vi "zc_jy.vi"(0 "action":string, 1 "LabVIEW Web Service Request":refnum<class "Web Request.lvclass"> caption="LabVIEW Web服务请求", 2 "jsren":string, 3 "sp_yijian":string, 5 "id":string, 7 "zc_luodi_num":string, 8 "sp_shuoming":string, 9 "zhriqi":string, 11 "didian":string, 12 "yongtu":string, 13 "shuoming":string, 14 "lc_num":string, 15 "key":string) -> (4 "error":errorcluster)   [LabVIEW 2017]
uses:
  <vilib>/wsapi/Web Request.lvclass
panel:
  in  "error 3":errorcluster={"status"=TRUE, "code"=255, "source"="当前资产不是“入库”状态！"} caption="error"
  out "postdata":string caption="post数据"
  out "error out":errorcluster caption="错误输出"
  # "Web服务请求输入接线端用于调用“Web服务”选板的VI。除非不需要访问该选板，否则不要在连线板上删除这个输入接线端。"
  # "添加至连线板的每一个其他输入控件，在URL中对应于一个输入。如需在接线端模式输出（默认设置）下包含显示控件，则该显示控件必须与连线板相连。"
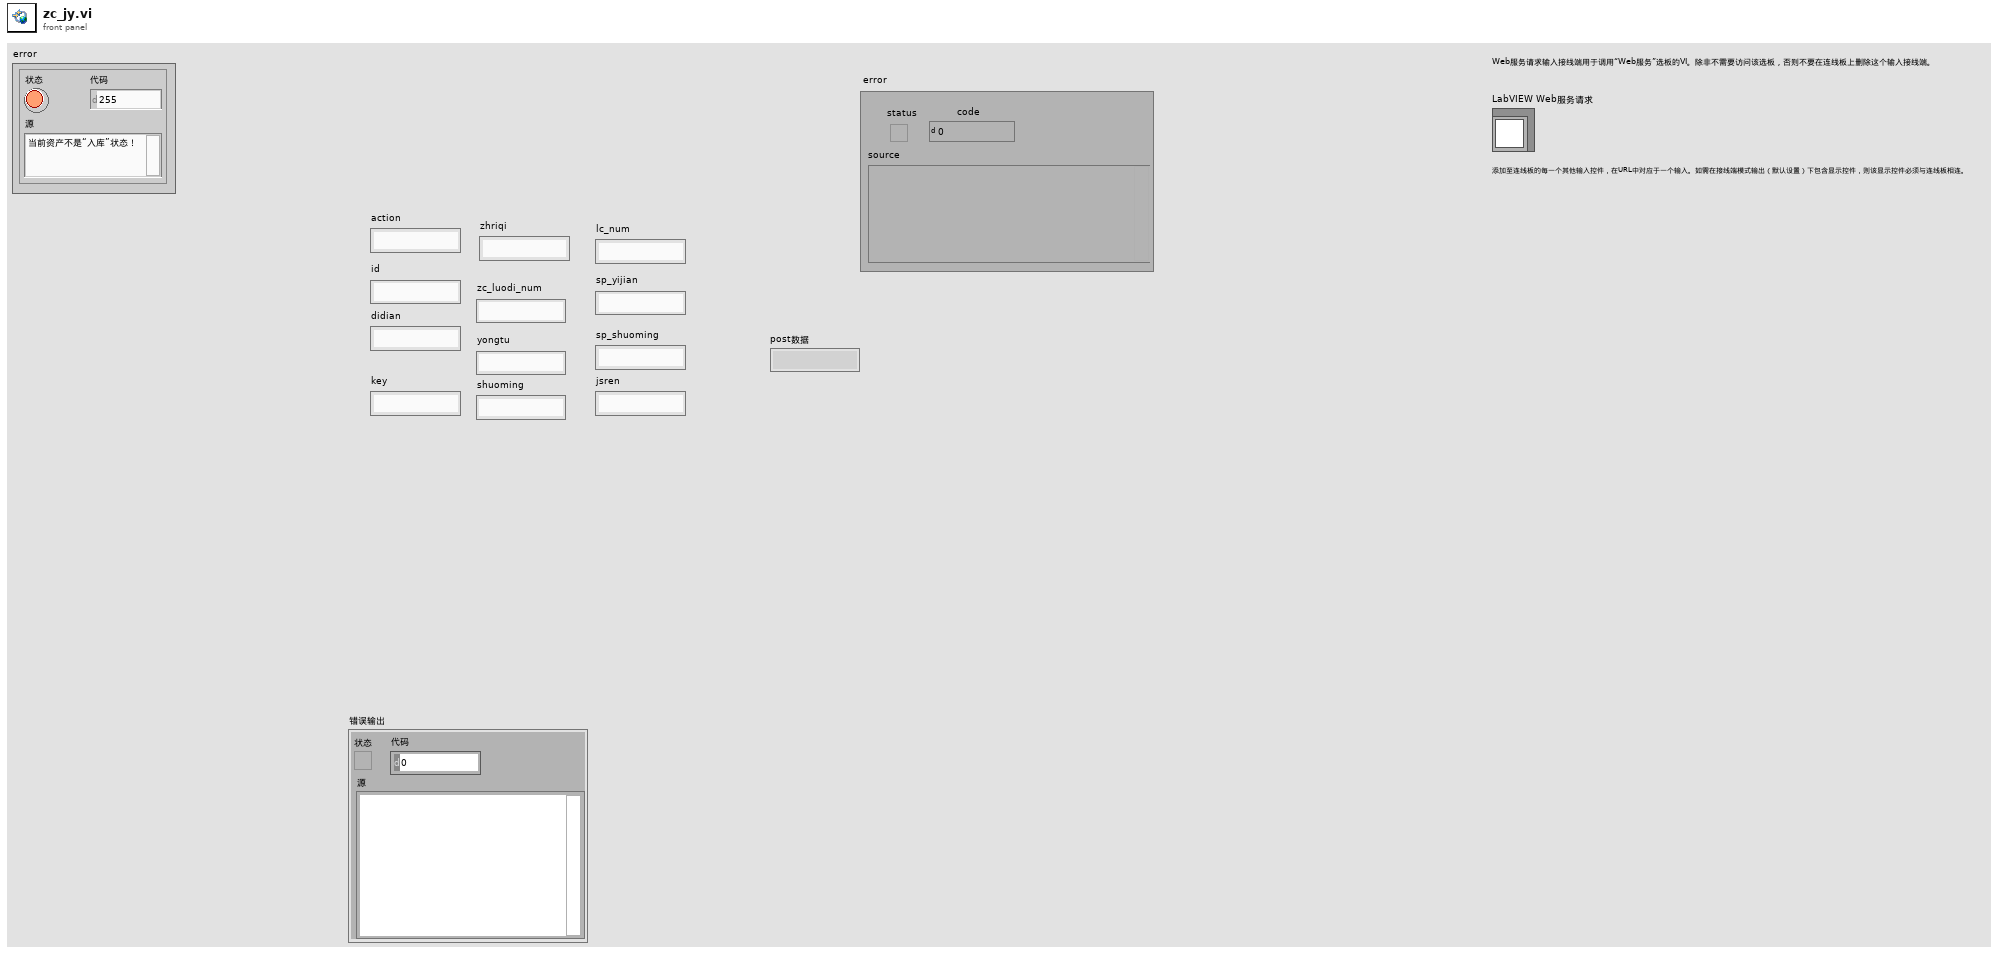
[diagram p1: front panel]
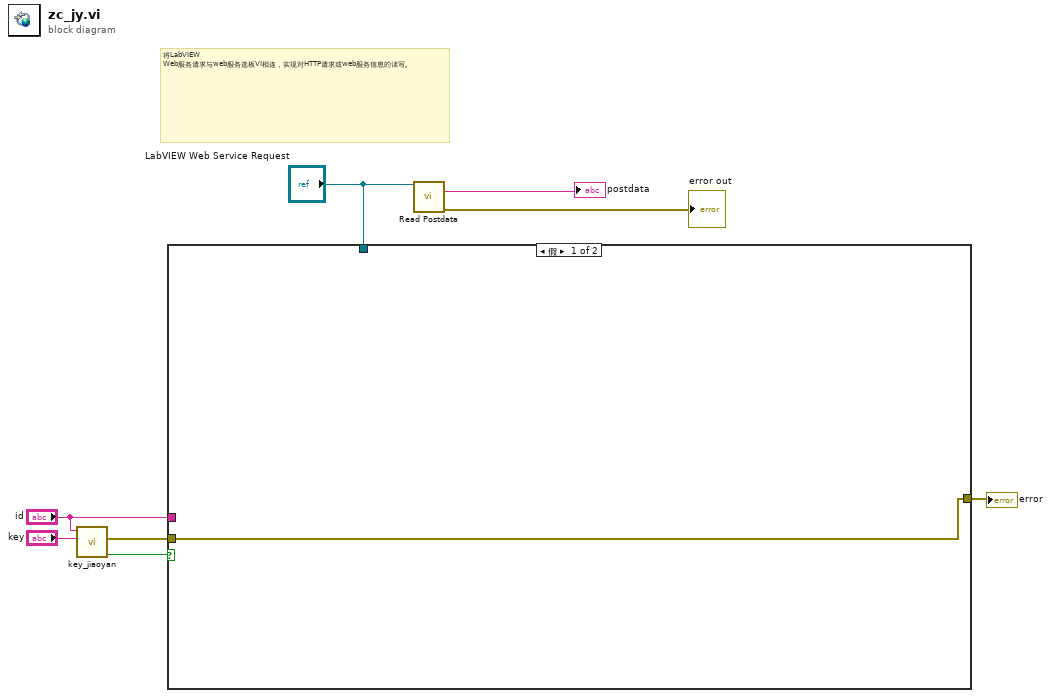
[diagram p0: block diagram]
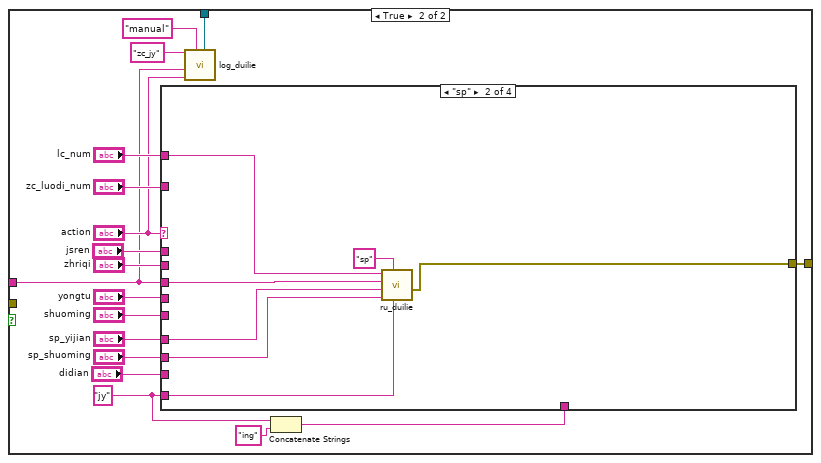
[diagram p2: hidden frame]
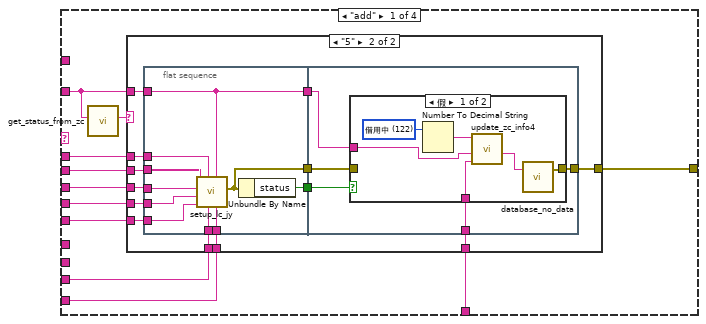
[diagram p3: hidden frame]
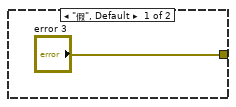
[diagram p4: hidden frame]
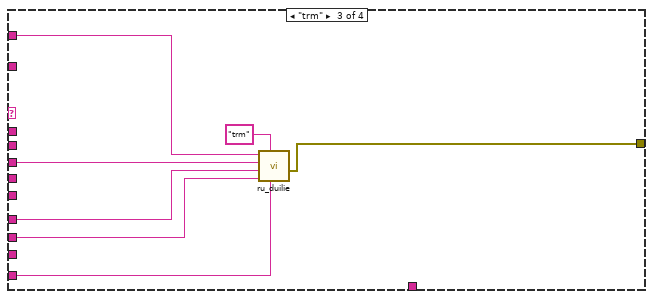
[diagram p6: hidden frame]
diagram:
  # "将LabVIEW Web服务请求与web服务选板VI相连，实现对HTTP请求或web服务信息的读写。"
  n1 = call "key_jiaoyan.vi"("key_client"="key", "gonghao"="id") -> ("jy"=w2:bool, "error"=w1:errorcluster)  [unwired: 8 in]
  n2 = case shown="假" w2 {
    tunnel: [w9 w20] -> w7
    tunnel: "LabVIEW Web Service Request" -> [_ w12]
    tunnel: "id" -> [_ w10]
    tunnel: w1 -> [w9 _]
    frame False {
    }
    frame True {
      w18 = "jy" ("yw")
      n3 = call "log_duilie.vi"("LabVIEW Web Service Request"=w12, "type"="manual", "action"="action", "user"=w10, "yw"="zc_jy") -> ()  [unwired: 7 in]
      n4 = Concatenate Strings(w18, "ing" ("字符串")) -> (w17:string)
      n5 = case shown="\"sp\"" "action" {
        tunnel: w10 -> [w35 w80 w87 _]
        tunnel: "zc_luodi_num" -> [w29 _ _ _]
        tunnel: "lc_num" -> [_ w79 w86 _]
        tunnel: "sp_yijian" -> [_ w78 w85 _]
        tunnel: "sp_shuoming" -> [_ w77 w84 _]
        tunnel: "zhriqi" -> [w38 _ _ _]
        tunnel: w18 -> [w34 w76 w83 _]
        tunnel: "yongtu" -> [w37 _ _ _]
        tunnel: "shuoming" -> [w36 _ _ _]
        tunnel: [w33 w75 w82 _] -> w20
        tunnel: w17 -> [w32 _ _ _]
        tunnel: "didian" -> [w31 _ _ _]
        tunnel: "jsren" -> [w30 _ _ _]
        frame "add" {
          n6 = call "get_status_from_zc.vi"("zc_luodi_num"=w29) -> ("status"=w28:string)  [unwired: 9 in, 1 out]
          n7 = case shown="\"5\"" w28 {
            tunnel: w38 -> [_ w51]
            tunnel: w37 -> [_ w50]
            tunnel: w36 -> [_ w49]
            tunnel: w35 -> [_ w48]
            tunnel: w34 -> [_ w47]
            tunnel: ["error 3" w46] -> w33
            tunnel: w32 -> [_ w45]
            tunnel: w31 -> [_ w44]
            tunnel: w30 -> [_ w43]
            tunnel: w29 -> [_ w42]
            frame "假", Default {
            }
            frame "5" {
              n8 = flat-sequence {
                tunnel: w42 -> [w56]
                tunnel: w50 -> [w60]
                tunnel: w49 -> [w59]
                tunnel: w51 -> [w62]
                tunnel: w48 -> [w61]
                tunnel: w47 -> [w57]
                tunnel: [w56] -> w52
                tunnel: w44 -> [w58]
                tunnel: w43 -> [w55]
                tunnel: [w54] -> w41
                tunnel: [w53] -> w40
                tunnel: w52 -> [w65]
                tunnel: [w67] -> w46
                tunnel: w45 -> [w66]
                tunnel: w41 -> [w64]
                tunnel: w40 -> [w63]
                frame #0 {
                  n9 = call "setup_lc_jy.vi"("yw"=w57, "zc_luodi_num"=w56, "didian"=w58, "jsren"=w55, "shuoming"=w59, "yongtu"=w60, "id"=w61, "zhriqi"=w62) -> ("error"=w53:errorcluster)  [unwired: 3 in]
                  n10 = Unbundle By Name(w53) -> ("status"=w54:bool)
                }
                frame #1 {
                  n11 = case shown="假" w64 {
                    tunnel: [w71 w74] -> w67
                    tunnel: w66 -> [w70 _]
                    tunnel: w65 -> [w68 _]
                    tunnel: w63 -> [_ w74]
                    frame False {
                      w69 = u8 122 items=["待验收"=1, "无需验收"=2, "验收不合格"=3, "待入库"=4, "入库"=5, "领用"=6, "借用"=7, "托管"=8, "接管"=9, "退出"=10, "出库在用"=11, "盘亏"=12, "出售"=13, "报废"=14, "领用中"=120, "退库中"=121, "借用中"=122, "归还中"=123, "转移中"=124, "调拨中"=125, "借调中"=126, "托管中"=127, "终止托管中"=128, "退出中"=129, "处置中"=130] ("状态选择器")
                      n12 = Number To Decimal String(number=w69) -> (decimal integer string=w72:string)  [unwired: 1 in]
                      n13 = call "update_zc_info4.vi"("ywxinxi"=w70, "number"=w68, "status"=w72) -> ("data_str"=w73:string)  [unwired: 8 in]
                      n14 = call "database_no_data.vi"("input"=w73) -> ("error"=w71:errorcluster)  [unwired: 2 in]
                    }
                    frame True {
                    }
                  }
                }
              }
            }
          }
        }
        frame "sp" {
          n15 = call "ru_duilie.vi"("yw"=w76, "name"="sp" ("元素"), "sp_shuoming"=w77, "sp_yijian"=w78, "id"=w80, "lc_num"=w79) -> ("error"=w75:errorcluster)  [unwired: 5 in]
        }
        frame "trm" {
          n16 = call "ru_duilie.vi"("yw"=w83, "name"="trm" ("元素"), "sp_shuoming"=w84, "sp_yijian"=w85, "id"=w87, "lc_num"=w86) -> ("error"=w82:errorcluster)  [unwired: 5 in]
        }
        frame Default {
        }
      }
    }
  }
  "error" <- w7
  n17 = call <vilib>:"Read Postdata.vi"("LabVIEW Web Service Request"="LabVIEW Web Service Request") -> ("postdata"=→"postdata":string, "error out"=→"error out":errorcluster)  [unwired: 12 in, 1 out]
